vi "SVFA Power Spectral Density (N Ch).vi"(0 "scaled signals [EU]":waveform(dbl)[](array[waveform]), 2 "window":T8=1 items=["None"=0, "Hanning"=1, "Hamming"=2, "Blackman-Harris"=3, "Exact Blackman"=4, "Blackman"=5, "Flat Top"=6, "4 Term B-Harris "=7, "7 Term B-Harris"=8, "Low Sidelobe"=9, "Force"=64, "Exponential"=65, "Blackman Nuttall"=11, "Triangle"=30, "Bartlett-Hanning"=31, "Bohman"=32, "Parzen"=33, "Welch"=34, "Kaiser"=60, "Dolph-Chebyshev"=61, "Gaussian"=62], 4 "dB On (F)":bool, 5 "error in (no error)":errorcluster, 6 "desired units":enum16{"EU^2 / Hz", "EU / sqrt(Hz)"}(ring), 7 "averaging parameters":T7={"averaging mode"=enum."No averaging", "weighting mode"=enum."Exponential", "number of averages"=10, "linear mode"=enum."One shot"} {"number of averages" min=1 step=1}, 9 "restart averaging (F)":bool) -> (11 "averaging done":bool, 13 "averages completed":dbl, 14 "power spectral densities [EU^2 rms / Hz]":cluster{"f0":dbl, "df":dbl, "magnitude":dbl[]}[](array[cluster]) {"magnitude" format="%.2p"; "df" format="%.2p"; "f0" format="%.2p"}, 15 "unit labels":string[](array[string]), 18 "spectrum info":T1[](array[typedef]) {"x-axis units" items=["Time (s)"=0, "Frequency-CB (Hz)"=1, "Frequency-CPB (Hz)"=1248, "Frequency-Arbitrary (Hz)"=2357, "Quefrency (s)"=2, "Revolutions (rev)"=3, "Order"=4, "Speed (RPM)"=11, "Speed (rad/s)"=21, "Index"=65535]; "weighting filter" items=["Linear", "A-weighting", "B-weighting", "C-weighting", "ITU-R 468-4", "Dolby", "CCITT", "C-message", "Wb", "Wc", "Wd", "We", "Wf", "Wh", "Wj", "Wk", "Wm", "AES17 20 kHz lowpass", "AES17 40 kHz lowpass", "AES17 20 kHz highpass", "AES17 40 kHz highpass"]; "dB reference [EU]" format="%.2f"; "engineering units" items=["custom..."=0, "V"=1, "A"=21, "C"=30, "pC"=31, "s"=32, "-"=29, "Pa"=2, "N"=20, "g"=3, "m/s^2"=4, "m/s"=5, "m"=6, "mm/s"=12, "mm"=13, "micron/s"=14, "micron"=15, "in/s^2"=7, "in/s"=8, "in"=9, "mil/s"=10, "mil"=11, "rad/s^2"=16, "rad/s"=17, "rad"=18, "deg/s^2"=26, "deg/s"=27, "deg"=28, "RPM"=22, "cycle/s^2"=23, "Hz"=24, "cycle"=25, "strain"=19]; "spectral info"."window" items=["None "=0, "Hanning"=1, "Hamming"=2, "Blackman-Harris"=3, "Exact Blackman"=4, "Blackman"=5, "Flat Top"=6, "4 Term B-Harris "=7, "7 Term B-Harris"=8, "Low Sidelobe"=9, "Force - Exponential"=10, "Gaussian"=62]}, 19 "error out":errorcluster)   [LabVIEW 2017]
doc: "Computes the power spectral density of <B>scaled signal [EU]</B> and returns the result in the selected units. Use the power spectral density to make repeatable measurements of the noise floor that are independent of the block size. Wire data to the <B>scaled signal [EU]</B> input to determine the polymorphic instance to use or manually select the instance."
uses:
  <vilib>/addons/_NISVFA/_Shared subVIs/Controls/svc_Window.ctl
  <vilib>/addons/_NISVFA/_Shared subVIs/Controls/svc_Spectrum Info.ctl
  <vilib>/addons/_NISVFA/_Shared subVIs/Controls/svc_X-Axis Units.ctl
  <vilib>/addons/_NISVFA/_Shared subVIs/Controls/svc_Spectrum Type.ctl
  <vilib>/addons/_NISVFA/_Shared subVIs/Controls/svc_Engineering Units Text Ring.ctl
  <vilib>/addons/_NISVFA/_Shared subVIs/Controls/svc_Weighting Filter Text Ring.ctl
  <vilib>/addons/_NISVFA/_Shared subVIs/Controls/svc_Complimentary Spectrum Units.ctl
  <vilib>/Analysis/2dsp.llb/Power Spectrum (DBL).vi
  <vilib>/Analysis/2dsp.llb/Real FFT.vi
  <vilib>/addons/_NISVFA/_Shared subVIs/Windowing/svfa_Scaled Time Domain Window (1 Ch).vi
  <vilib>/addons/_NISVFA/_Shared subVIs/Spectrum Info/svfa_Build Spectrum Info.vi
  <vilib>/addons/_NISVFA/_Shared subVIs/Spectrum Averaging/svfa_No Average Array (complex).vi
  <vilib>/addons/_NISVFA/_Shared subVIs/Spectrum Averaging/svfa_Average Array (complex).vi
  <vilib>/addons/_NISVFA/_Spectrum Processing/subVIs/svfa_Peak to RMS to Peak2Peak.vi
  <vilib>/addons/_NISVFA/_Spectrum Processing/subVIs/svfa_Mag to Mag2.vi
  <vilib>/addons/_NISVFA/_Spectrum Processing/subVIs/svfa_Linear to dB.vi
  <vilib>/addons/_NISVFA/_Spectrum Processing/subVIs/svfa_dBrefA to dBrefB.vi
  <vilib>/addons/_NISVFA/_Spectrum Processing/subVIs/svfa_Spectrum to Spectral Density.vi
  <vilib>/addons/_NISVFA/_Shared subVIs/Windowing/svfa_Scaled Time Domain Window (Array).vi
  <vilib>/addons/_NISVFA/_Shared subVIs/Common/svc_Get SV Channel Info.vi
  <vilib>/Analysis/4window.llb/Force Window.vi
  <vilib>/Analysis/4window.llb/Force Window (DBL).vi
  <vilib>/Analysis/4window.llb/Exponential Window.vi
  <vilib>/Analysis/4window.llb/Exponential Window (DBL).vi
  <vilib>/addons/_NISVFA/_Shared subVIs/Common/svc_Get Weighting Enum and Labels.vi
  <vilib>/addons/_NISVFA/_Shared subVIs/Common/svc_Unit Label Lexical Class.vi
  <vilib>/addons/_NISVFA/_Shared subVIs/Common/svc_Engineering Units to Unit Label.vi
  <vilib>/addons/_NISVFA/_Shared subVIs/Common/svc_Format Value (DBL).vi
  <vilib>/addons/_NISVFA/_Shared subVIs/Common/svc_Window Parameters.vi
  <vilib>/Utility/error.llb/Error Cluster From Error Code.vi
  <vilib>/Analysis/0measdsp.llb/Scaled Time Domain Window.vi
  <vilib>/Analysis/0measdsp.llb/Scaled Time Domain Window (DBL).vi
  <vilib>/addons/_NISVFA/_Spectrum Processing/subVIs/svfa_Spectrum Info Window to windowTd Type Def.vi
  <vilib>/addons/_NISVFA/_Shared subVIs/Common/svc_Get Window Info.vi
  <vilib>/addons/_NISVFA/_Shared subVIs/Common/svc_Channel Info to Spectrum Info.vi
  <vilib>/addons/_NISVFA/_Shared subVIs/Common/svc_Unit Label to Engineering Units.vi
  <vilib>/Analysis/NI_AALPro.lvlib
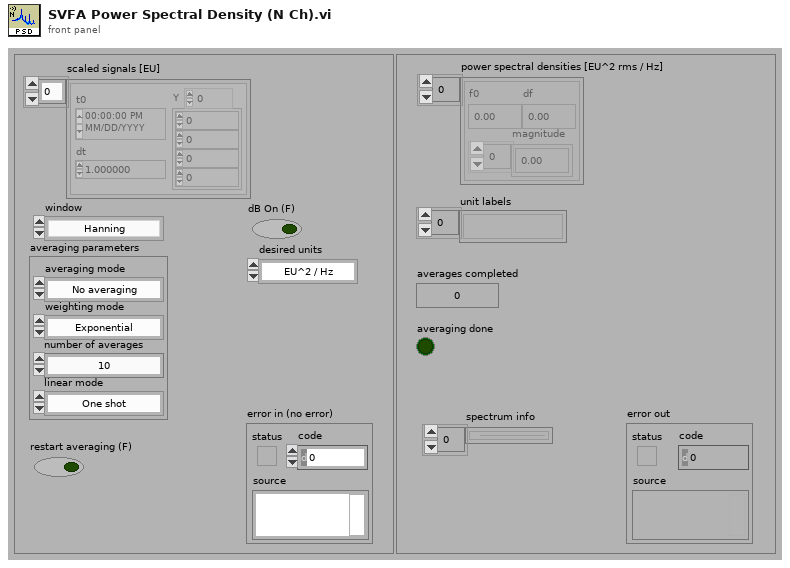
[diagram p1: front panel]
types:
  T1 = typedef "svc_Spectrum Info.ctl" = cluster{"channel name":string, "description":string, "x-axis units":T2, "spectral info":cluster{"spectrum type":T3, "linear/dB":enum16{"linear", "dB"}, "window":u16, "window size":i32, "FFT size":i32}, "engineering units":T4, "custom label":string, "dB reference [EU]":dbl, "peak units":enum16{"rms", "peak", "peak-peak"}, "weighting filter":T5, "spectral density?":bool, "unit label":string, "spectrum skewed?":bool, "complimentary spectrum units":T6}
  T2 = typedef "svc_X-Axis Units.ctl" = u16
  T3 = typedef "svc_Spectrum Type.ctl" = enum16{"FFT Spectrum [complex]", "Amplitude [Magnitude]", "Power [Magnitude^2]", "Cross Spectrum [complex]", "Frequency Response [Complex]"}
  T4 = typedef "svc_Engineering Units Text Ring.ctl" = u16
  T5 = typedef "svc_Weighting Filter Text Ring.ctl" = u16
  T6 = typedef "svc_Complimentary Spectrum Units.ctl" = enum16{"none", "radians", "degrees", "cycles", "imaginary"}
  T7 = cluster{"averaging mode":enum16{"No averaging", "Vector averaging", "RMS averaging", "Peak hold"}, "weighting mode":enum16{"Linear", "Exponential"}, "number of averages":u32, "linear mode":enum16{"One shot", "Auto restart"}}
  T8 = typedef "svc_Window.ctl" = u32
  T9 = cluster{"linear/dB":enum16{"no change", "linear", "dB"}, "dB reference (0: no change)":dbl, "power/magnitude":enum16{"no change", "power", "magnitude"}, "view":enum16{"no change", "rms", "peak", "peak-peak"}}
  T10 = enum16{"Restart processing", "Continue processing", "Skip processing"}
  T11 = enum16{"no change", "spectrum", "spectral density"}
  T12 = cluster{"complex FFT":cdb[], "real FFT":dbl[], "f0":dbl, "df":dbl, "averages completed":dbl, "averaging parameters":cluster{"averaging mode":enum16{"No averaging", "Vector averaging", "RMS averaging", "Peak hold"}, "weighting mode":enum16{"Linear", "Exponential"}, "number of averages":u32, "linear mode":enum16{"One shot", "Auto restart"}}}[]
  T13 = enum16{"No averaging", "Vector averaging", "RMS averaging", "Peak hold"}
  T14 = cluster{"complex FFT":cdb[], "real FFT":dbl[], "f0":dbl, "df":dbl, "averages completed":dbl, "averaging parameters":cluster{"averaging mode":enum16{"No averaging", "Vector averaging", "RMS averaging", "Peak hold"}, "weighting mode":enum16{"Linear", "Exponential"}, "number of averages":u32, "linear mode":enum16{"One shot", "Auto restart"}}}
  T15 = cluster{"complex FFT":cdb[], "Mag/Real FFT":dbl[], "f0":dbl, "df":dbl, "averages completed":dbl, "averaging parameters":cluster{"averaging mode":enum16{"No averaging", "Vector averaging", "RMS averaging", "Peak hold"}, "weighting mode":enum16{"Linear", "Exponential"}, "number of averages":u32, "linear mode":enum16{"One shot", "Auto restart"}}}
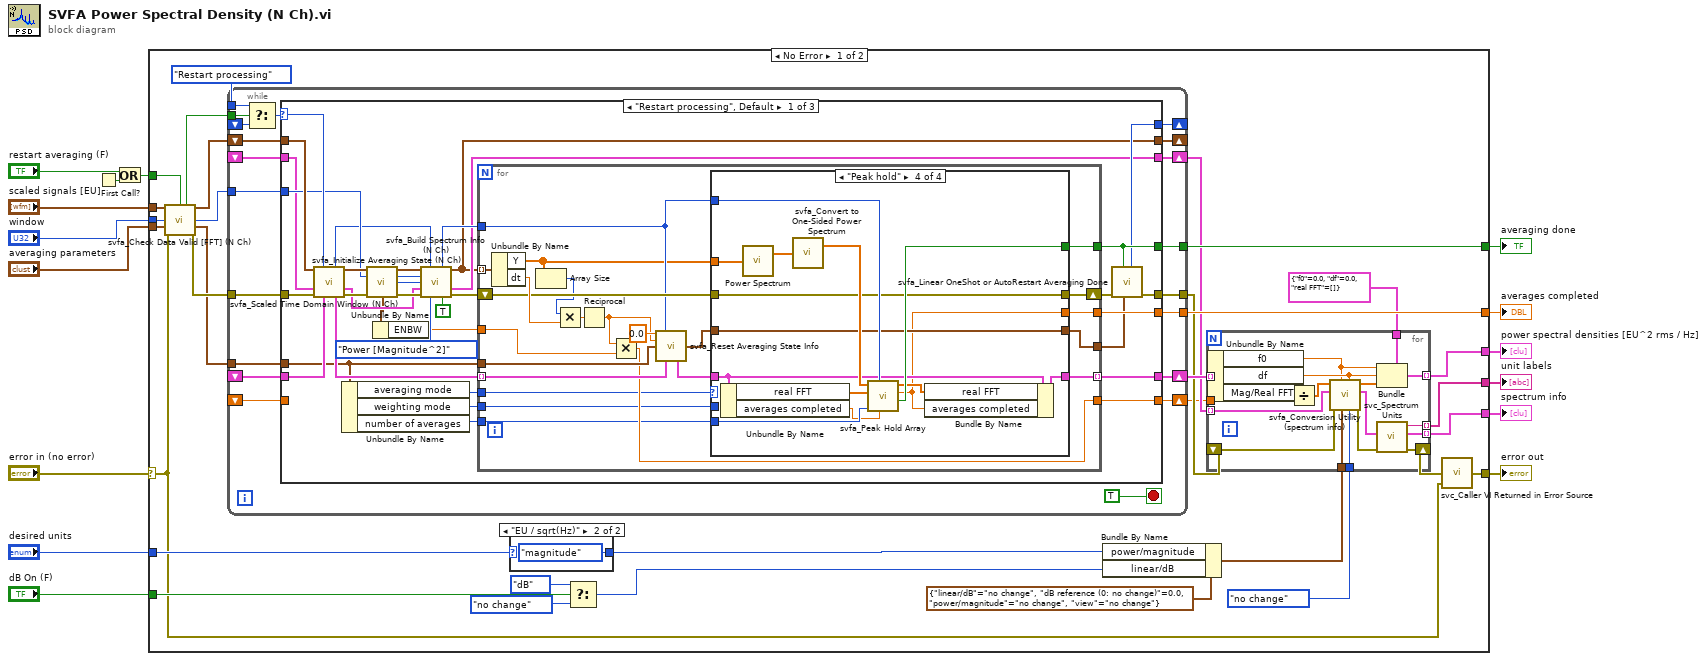
[diagram p0: block diagram]
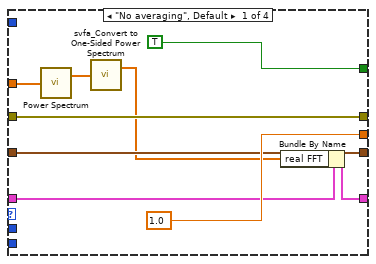
[diagram p2: hidden frame]
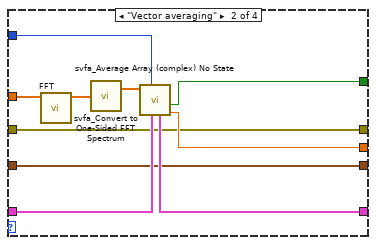
[diagram p3: hidden frame]
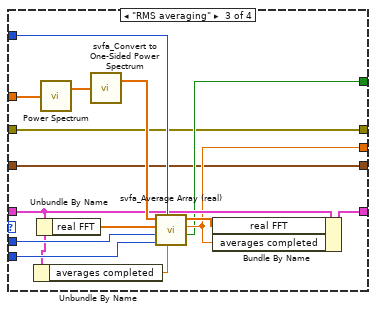
[diagram p4: hidden frame]
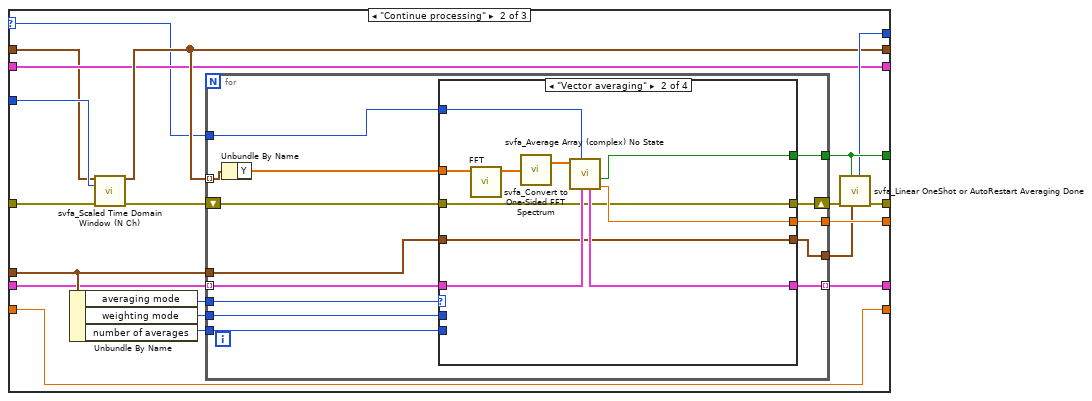
[diagram p5: hidden frame]
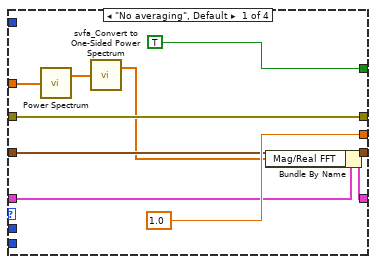
[diagram p6: hidden frame]
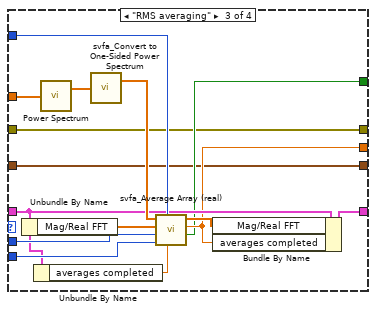
[diagram p7: hidden frame]
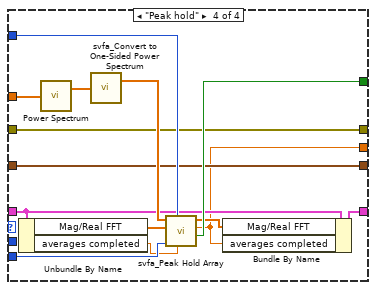
[diagram p8: hidden frame]
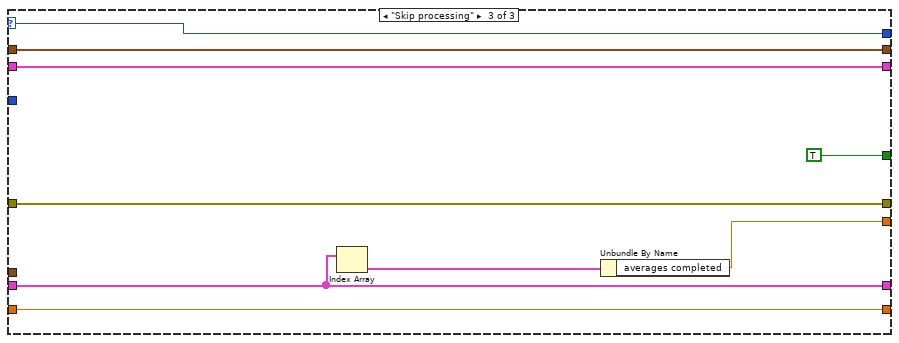
[diagram p9: hidden frame]
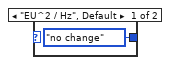
[diagram p10: hidden frame]
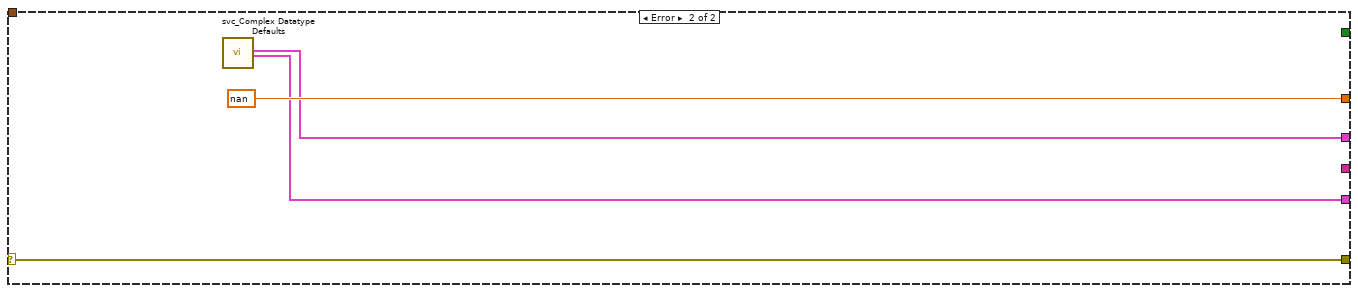
[diagram p11: hidden frame]
diagram:
  n1 = First Call?() -> (First Call?: T/F=w4:bool)
  n2 = Or(x="restart averaging (F)", y=w4) -> (x .or. y?=w2:bool)
  n3 = case shown="No Error" "error in (no error)" {
    selector: "error in (no error)" -> [w40 w287]
    tunnel: "scaled signals [EU]" -> [w46 _]
    tunnel: w2 -> [w45 _]
    tunnel: [w42 w287] -> w13
    tunnel: [w18 w286] -> w12
    tunnel: [w27 _] -> w11
    tunnel: [w26 nan ("averages completed")] -> w10
    tunnel: "dB On (F)" -> [w47 _]
    tunnel: [w22 _] -> w8
    tunnel: [w19 w285] -> w7
    tunnel: "window" -> [w44 _]
    tunnel: "averaging parameters" -> [w43 _]
    tunnel: "desired units" -> [w41 _]
    frame No Error {
      n4 = call <vilib>:"svfa_Check Data Valid [FFT] (N Ch).vi"("scaled signals"=w46, "restart averaging (F)"=w45, "window"=w44, "averaging parameters"=w43, "error in (no error)"=w40) -> ("restart averaging"=w32:bool, "dup scaled signals"=w31:waveform(dbl)[], "dup window"=w29:T8, "dup averaging parameters"=w28:T7, "error out"=w30:errorcluster)  [unwired: 6 in]
      n5 = while {
        tunnel: w29 -> [w76]
        tunnel: [w77] -> w26
        tunnel: [w78] -> w27
        tunnel: w28 -> [w79]
        tunnel: [w80] -> w21
        shift-left: _ -> [w81]
        shift-right: [w82] -> w33
        tunnel: w30 -> [w84]
        shift-right: [w75] -> w17
        shift-left: _ -> [w74]
        shift-right: [w73] -> _
        shift-left: _ -> [w72]
        tunnel: w32 -> [w70]
        tunnel: T10."Restart processing" ("t") -> [w69]
        shift-right: [w68] -> _
        shift-left: w31 -> [w83]
        shift-right: [w67] -> w16
        shift-left: _ -> [w66]
        stop <- TRUE stop-if-true
        n6 = Select(t=w69, s=w70, f=w72) -> (s? t:f=w71:T10)
        n7 = case shown="\"Restart processing\", Default" w71 {
          selector: w71 -> [w111 w195 w275]
          tunnel: w84 -> [w113 w197 w278]
          tunnel: w83 -> [w117 w193 w276]
          tunnel: [w119 w210 w277] -> w82
          tunnel: w81 -> [w115 w194 w277]
          tunnel: [w104 w202 w278] -> w80
          tunnel: w79 -> [w108 w206 _]
          tunnel: [w109 w207 TRUE ("averaging done")] -> w78
          tunnel: [w118 w209 w280] -> w77
          tunnel: w76 -> [w110 w208 _]
          tunnel: [w94 w198 w279] -> w75
          tunnel: w74 -> [w97 w198 w279]
          tunnel: [w106 w204 w275] -> w73
          tunnel: [w93 w199 w276] -> w68
          tunnel: [w88 w192 w274] -> w67
          tunnel: w66 -> [_ w192 w274]
          frame "Restart processing", Default {
            n8 = call <vilib>:"svfa_Initialize Averaging State (N Ch).vi"("Windowed Waveform(s)"=w117, "processing control in"=w111, "spectra info in"=w97, "error in (no error)"=w113, "state info"=w115) -> ("processing control out"=w95:T10, "Windowed Waveform(s)"=w116:waveform(dbl)[], "spectra info out"=w96:T1[], "state info"=w114:T12, "error out"=w112:errorcluster)  [unwired: 6 in]
            n9 = Unbundle By Name(w108) -> ("averaging mode"=w120:T13, "weighting mode"=w87:enum16{"Linear", "Exponential"}, "number of averages"=w86:u32)
            n10 = call <vilib>:"svfa_Scaled Time Domain Window (N Ch).vi"("Scaled signal(s)"=w116, "window"=w110, "error in (no error)"=w112) -> ("Windowed Waveform(s)"=w103:waveform(dbl)[], "window"=w102:T8, "window length"=w89:i32, "window constants"=w91:cluster{"ENBW":dbl, "CG":dbl}, "error out"=w101:errorcluster)  [unwired: 8 in]
            n11 = Unbundle By Name(w91) -> ("ENBW"=w90:dbl)
            n12 = call <vilib>:"svfa_Build Spectrum Info (N Ch).vi"("scaled signal(s)"=w103, "processing control in"=w95, "window"=w102, "window size"=w89, "spectra info in"=w96, "error in (no error)"=w101, "spectrum type"=svc_Spectrum_Type."Power [Magnitude^2]", "spectral density?"=TRUE) -> ("dup processing control"=w99:T10, "dup scaled signals"=w93:waveform(dbl)[], "spectra info out"=w94:T1[], "error out"=w100:errorcluster)  [unwired: 4 in]
            n13 = for {
              tunnel: [w131] -> w119 mode=indexing
              tunnel: [w128] -> w109
              tunnel: [w123] -> w118
              tunnel: w120 -> [w124]
              tunnel: w114 -> [w141] mode=indexing
              tunnel: w108 -> [w140]
              tunnel: w99 -> [w127]
              tunnel: [w132] -> w107
              tunnel: w93 -> [w143] mode=indexing
              shift-right: [w129] -> w105
              shift-left: w100 -> [w130]
              tunnel: w90 -> [w142]
              tunnel: [w135] -> w88
              tunnel: w87 -> [w126]
              tunnel: w86 -> [w125]
              n14 = Unbundle By Name ("Get Waveform Components")(w143) -> ("Y"=w122:dbl[], "dt"=w137:dbl)
              n15 = Array Size(array=w122) -> (size(s)=w121:i32)
              n16 = Multiply(x=w121, y=w137) -> (x*y=w138:dbl)
              n17 = Reciprocal(x=w138) -> (1/x=w136:dbl)
              n18 = Multiply(x=w136, y=w142) -> (x*y=w135:dbl)
              n19 = call <vilib>:"svfa_Reset Averaging State Info.vi"("f0"=0.0, "processing control"=w127, "df"=w136, "averaging parameters"=w140, "averaging state info in"=w141) -> ("dup averaging parameters"=w133:T7, "averaging state info out"=w134:T14)  [unwired: 9 in]
              n20 = case shown="\"Peak hold\"" w124 {
                tunnel: [w148 w153 w163 w183] -> w129
                tunnel: [1.0 ("averages completed") w161 w166 w178] -> w123
                tunnel: [TRUE ("averaging done") w155 w165 w186] -> w128
                tunnel: w130 -> [w148 w153 w163 w183]
                tunnel: w133 -> [w147 w154 w164 w182]
                tunnel: w127 -> [_ w162 w170 w189]
                tunnel: w122 -> [w149 w159 w176 w190]
                tunnel: [w145 w156 w171 w179] -> w131
                tunnel: w134 -> [w146 w160 w168 w180]
                tunnel: w126 -> [_ _ w175 _]
                tunnel: w125 -> [_ _ w174 w187]
                tunnel: [w147 w154 w164 w182] -> w132
                frame "No averaging", Default {
                  n21 = call-poly <vilib>:"Power Spectrum.vi"("X"=w149) -> ("Power Spectrum"=w150:dbl[])  [unwired: 1 out]
                  n22 = call <vilib>:"svfa_Convert to One-Sided Power Spectrum.vi"("two-sided power spectrum"=w150) -> ("one-sided power spectrum"=w144:dbl[])  [unwired: 1 out]
                  n23 = Bundle By Name(cluster=w146, "real FFT"=w144) -> (w145:T14)
                }
                frame "Vector averaging" {
                  n24 = call-poly <vilib>:"FFT.vi"("X"=w159) -> ("FFT {X}"=w158:cdb[])  [unwired: 9 in, 1 out]
                  n25 = call <vilib>:"svfa_Convert to One-Sided FFT Spectrum.vi"("two-sided FFT spectrum"=w158) -> ("one-sided FFT spectrum"=w157:cdb[])  [unwired: 1 out]
                  n26 = call <vilib>:"svfa_Average Array (complex) No State.vi"("averaging state info in"=w160, "processing control"=w162, "array"=w157) -> ("averages completed"=w161:dbl, "averaging done"=w155:bool, "averaging state info out"=w156:T15)  [unwired: 5 in, 1 out]
                }
                frame "RMS averaging" {
                  n27 = Unbundle By Name(w168) -> ("averages completed"=w169:dbl)
                  n28 = Unbundle By Name(w168) -> ("real FFT"=w172:dbl[])
                  n29 = call-poly <vilib>:"Power Spectrum.vi"("X"=w176) -> ("Power Spectrum"=w177:dbl[])  [unwired: 1 out]
                  n30 = call <vilib>:"svfa_Convert to One-Sided Power Spectrum.vi"("two-sided power spectrum"=w177) -> ("one-sided power spectrum"=w173:dbl[])  [unwired: 1 out]
                  n31 = call <vilib>:"svfa_Average Array (real).vi"("averages completed in"=w169, "processing control"=w170, "number of averages"=w174, "weighting mode"=w175, "previous average array"=w172, "array"=w173) -> ("averaging done"=w165:bool, "averages completed out"=w166:dbl, "average array"=w167:dbl[])  [unwired: 3 in]
                  n32 = Bundle By Name(cluster=w168, "real FFT"=w167, "averages completed"=w166) -> (w171:T14)
                }
                frame "Peak hold" {
                  n33 = Unbundle By Name(w180) -> ("real FFT"=w188:dbl[], "averages completed"=w181:dbl)
                  n34 = call-poly <vilib>:"Power Spectrum.vi"("X"=w190) -> ("Power Spectrum"=w191:dbl[])  [unwired: 1 out]
                  n35 = call <vilib>:"svfa_Convert to One-Sided Power Spectrum.vi"("two-sided power spectrum"=w191) -> ("one-sided power spectrum"=w185:dbl[])  [unwired: 1 out]
                  n36 = call <vilib>:"svfa_Peak Hold Array.vi"("averages completed in"=w181, "processing control"=w189, "number of averages"=w187, "previous peak array"=w188, "array"=w185) -> ("averaging done"=w186:bool, "averages completed out"=w178:dbl, "peak array"=w184:dbl[])  [unwired: 4 in]
                  n37 = Bundle By Name(cluster=w180, "real FFT"=w184, "averages completed"=w178) -> (w179:T14)
                }
              }
            }
            n38 = call <vilib>:"svfa_Linear OneShot or AutoRestart Averaging Done.vi"("averaging parameters"=w107, "averaging done"=w109, "error in (no error)"=w105) -> ("error out"=w104:errorcluster, "processing control"=w106:T10)  [unwired: 7 in]
          }
          frame "Continue processing" {
            n39 = Unbundle By Name(w206) -> ("averaging mode"=w211:T13, "weighting mode"=w201:enum16{"Linear", "Exponential"}, "number of averages"=w200:u32)
            n40 = call <vilib>:"svfa_Scaled Time Domain Window (N Ch).vi"("Scaled signal(s)"=w193, "window"=w208, "error in (no error)"=w197) -> ("Windowed Waveform(s)"=w199:waveform(dbl)[], "error out"=w196:errorcluster)  [unwired: 8 in, 3 out]
            n41 = for {
              tunnel: [w223] -> w210 mode=indexing
              tunnel: [w220] -> w207
              tunnel: [w214] -> w209
              tunnel: w211 -> [w215]
              tunnel: w194 -> [w212] mode=indexing
              tunnel: w206 -> [w213]
              tunnel: w195 -> [w219]
              tunnel: [w224] -> w205
              tunnel: w199 -> [w225] mode=indexing
              shift-right: [w221] -> w203
              shift-left: w196 -> [w222]
              tunnel: w201 -> [w217]
              tunnel: w200 -> [w216]
              n42 = Unbundle By Name ("Get Waveform Components")(w225) -> ("Y"=w218:dbl[])
              n43 = case shown="\"Vector averaging\"" w215 {
                tunnel: [w230 w235 w245 w265] -> w221
                tunnel: [1.0 ("averages completed") w243 w248 w260] -> w214
                tunnel: [TRUE ("averaging done") w237 w247 w268] -> w220
                tunnel: w222 -> [w230 w235 w245 w265]
                tunnel: w213 -> [w229 w236 w246 w264]
                tunnel: w219 -> [_ w244 w252 w271]
                tunnel: w218 -> [w231 w241 w258 w272]
                tunnel: [w227 w238 w253 w261] -> w223
                tunnel: w212 -> [w228 w242 w250 w262]
                tunnel: w217 -> [_ _ w257 _]
                tunnel: w216 -> [_ _ w256 w269]
                tunnel: [w229 w236 w246 w264] -> w224
                frame "No averaging", Default {
                  n44 = call-poly <vilib>:"Power Spectrum.vi"("X"=w231) -> ("Power Spectrum"=w232:dbl[])  [unwired: 1 out]
                  n45 = call <vilib>:"svfa_Convert to One-Sided Power Spectrum.vi"("two-sided power spectrum"=w232) -> ("one-sided power spectrum"=w226:dbl[])  [unwired: 1 out]
                  n46 = Bundle By Name(cluster=w228, "Mag/Real FFT"=w226) -> (w227:T15)
                }
                frame "Vector averaging" {
                  n47 = call-poly <vilib>:"FFT.vi"("X"=w241) -> ("FFT {X}"=w240:cdb[])  [unwired: 9 in, 1 out]
                  n48 = call <vilib>:"svfa_Convert to One-Sided FFT Spectrum.vi"("two-sided FFT spectrum"=w240) -> ("one-sided FFT spectrum"=w239:cdb[])  [unwired: 1 out]
                  n49 = call <vilib>:"svfa_Average Array (complex) No State.vi"("averaging state info in"=w242, "processing control"=w244, "array"=w239) -> ("averages completed"=w243:dbl, "averaging done"=w237:bool, "averaging state info out"=w238:T15)  [unwired: 5 in, 1 out]
                }
                frame "RMS averaging" {
                  n50 = Unbundle By Name(w250) -> ("Mag/Real FFT"=w254:dbl[])
                  n51 = Unbundle By Name(w250) -> ("averages completed"=w251:dbl)
                  n52 = call-poly <vilib>:"Power Spectrum.vi"("X"=w258) -> ("Power Spectrum"=w259:dbl[])  [unwired: 1 out]
                  n53 = call <vilib>:"svfa_Convert to One-Sided Power Spectrum.vi"("two-sided power spectrum"=w259) -> ("one-sided power spectrum"=w255:dbl[])  [unwired: 1 out]
                  n54 = call <vilib>:"svfa_Average Array (real).vi"("averages completed in"=w251, "processing control"=w252, "number of averages"=w256, "weighting mode"=w257, "previous average array"=w254, "array"=w255) -> ("averaging done"=w247:bool, "averages completed out"=w248:dbl, "average array"=w249:dbl[])  [unwired: 3 in]
                  n55 = Bundle By Name(cluster=w250, "Mag/Real FFT"=w249, "averages completed"=w248) -> (w253:T15)
                }
                frame "Peak hold" {
                  n56 = Unbundle By Name(w262) -> ("Mag/Real FFT"=w270:dbl[], "averages completed"=w263:dbl)
                  n57 = call-poly <vilib>:"Power Spectrum.vi"("X"=w272) -> ("Power Spectrum"=w273:dbl[])  [unwired: 1 out]
                  n58 = call <vilib>:"svfa_Convert to One-Sided Power Spectrum.vi"("two-sided power spectrum"=w273) -> ("one-sided power spectrum"=w267:dbl[])  [unwired: 1 out]
                  n59 = call <vilib>:"svfa_Peak Hold Array.vi"("averages completed in"=w263, "processing control"=w271, "number of averages"=w269, "previous peak array"=w270, "array"=w267) -> ("averaging done"=w268:bool, "averages completed out"=w260:dbl, "peak array"=w266:dbl[])  [unwired: 4 in]
                  n60 = Bundle By Name(cluster=w262, "Mag/Real FFT"=w266, "averages completed"=w260) -> (w261:T15)
                }
              }
            }
            n61 = call <vilib>:"svfa_Linear OneShot or AutoRestart Averaging Done.vi"("averaging parameters"=w205, "averaging done"=w207, "error in (no error)"=w203) -> ("error out"=w202:errorcluster, "processing control"=w204:T10)  [unwired: 7 in]
          }
          frame "Skip processing" {
            n62 = Index Array(array=w277) -> (element=w281:T15)  [unwired: 1 in]
            n63 = Unbundle By Name(w281) -> ("averages completed"=w280:dbl)
          }
        }
      }
      n64 = case shown="\"EU / sqrt(Hz)\"" w41 {
        tunnel: [enum16{"no change", "power", "magnitude"}."no change" ("power/magnitude") enum16{"no change", "power", "magnitude"}."magnitude" ("power/magnitude")] -> w39
        frame "EU^2 / Hz", Default {
        }
        frame "EU / sqrt(Hz)" {
        }
      }
      n65 = Select(t=enum16{"no change", "linear", "dB"}."dB" ("linear/dB"), s=w47, f=enum16{"no change", "linear", "dB"}."no change" ("linear/dB")) -> (s? t:f=w36:enum16{"no change", "linear", "dB"})
      n66 = Bundle By Name(cluster=T9 {"linear/dB"=enum."no change", "dB reference (0: no change)"=0.0, "power/magnitude"=enum."no change", "view"=enum."no change"} ("desired scaling"), "power/magnitude"=w39, "linear/dB"=w36) -> (w24:T9)
      n67 = for {
        tunnel: w33 -> [w65] mode=indexing
        tunnel: [w64] -> w18 mode=indexing
        tunnel: cluster{"f0":dbl, "df":dbl, "real FFT":dbl[]} {"f0"=0.0, "df"=0.0, "real FFT"=[]} ("cluster") -> [w63]
        tunnel: w24 -> [w57]
        tunnel: T11."no change" ("spectral density desired") -> [w56]
        tunnel: [w55] -> w22 mode=indexing
        shift-right: [w54] -> w20
        shift-left: w21 -> [w52]
        tunnel: [w53] -> w19 mode=indexing
        tunnel: w17 -> [w51] mode=indexing
        tunnel: w16 -> [w48]
        n68 = Unbundle By Name(w65) -> ("f0"=w58:dbl, "df"=w59:dbl, "Mag/Real FFT"=w50:dbl[])
        n69 = Divide(x=w50, y=w48) -> (x/y=w49:dbl[])
        n70 = call <vilib>:"svfa_Conversion Utility (spectrum info).vi"("spectral density desired"=w56, "dx"=w59, "desired scaling"=w57, "x0"=w58, "error in (no error)"=w52, "spectrum info in"=w51, "input signal"=w49) -> ("error out"=w62:errorcluster, "spectrum info out"=w61:T1, "converted signal"=w60:dbl[])  [unwired: 2 in]
        n71 = Bundle(cluster=w63, "f0"=w58, "df"=w59, "real FFT"=w60) -> (w64:cluster{"f0":dbl, "df":dbl, "real FFT":dbl[]})
        n72 = call <vilib>:"svc_Spectrum Units.vi"("error in (no error)"=w62, "spectrum info in"=w61) -> ("error out"=w54:errorcluster, "spectrum info out"=w53:T1, "unit label"=w55:string)  [unwired: 2 in, 1 out]
      }
      n73 = call <vilib>:"svc_Caller VI Returned in Error Source.vi"("warning input to caller"=w40, "error in (no error)"=w20) -> ("error out"=w42:errorcluster)  [unwired: 3 in]
    }
    frame Error {
      n74 = call <vilib>:"svc_Complex Datatype Defaults.vi"() -> ("empty array of spectra"=w286:cluster{"f0":dbl, "df":dbl, "magnitude":dbl[]}[], "empty array of spectrum info"=w285:T1[])  [unwired: 11 in, 7 out]
    }
  }
  "error out" <- w13
  "averaging done" <- w11
  "averages completed" <- w10
  "unit labels" <- w8
  "power spectral densities [EU^2 rms / Hz]" <- w12
  "spectrum info" <- w7
